vi "Plot Update Cursor 2D Graph.vi"(8 "Cursor XY":T1, 11 "_Graph":refnum<vi>) -> ()   [LabVIEW 2016]
uses:
  <vilib>/addons/Software Calibration Management/xSCM/Controls/TLU1D.ctl
  <vilib>/addons/Software Calibration Management/xSCM/SCM-API.lvlib
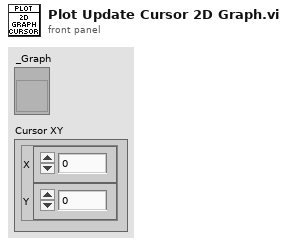
[diagram p1: front panel]
types:
  T1 = typedef "SCM-API.lvlib/TLU1D.ctl" = cluster{"X":sgl, "Y":sgl}
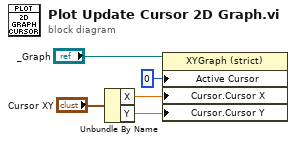
[diagram p0: block diagram]
diagram:
  n1 = Unbundle By Name("Cursor XY") -> ("X"=w3:sgl, "Y"=w2:sgl)
  n2 = property on="Property Node" class="XYGraph (strict)"(reference="_Graph", "Active Cursor"=u32 0, "Cursor.Cursor X"=w3, "Cursor.Cursor Y"=w2) -> ()  [unwired: 1 in, 2 out]
